vi "test_libssh2_userauth_publickey_fromfile.vi"() -> ()   [LabVIEW 2013, in "libssh2_integration_tests.lvlib"]
uses:
  libssh2_integration_tests.lvlib
  libssh2/libssh2_init_default.vi
  libssh2/libssh2_session_handshake_tcp.vi
  libssh2/libssh2.lvlib
  <vilib>/addons/_JKI Toolkits/Caraya/classes/Test/Test.lvclass
  <vilib>/addons/_JKI Toolkits/Caraya/classes/Assert/Assert.lvclass
panel:
  out "error out":errorcluster
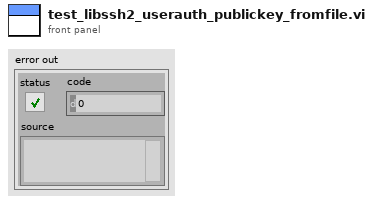
[diagram p1: front panel]
types:
  T1 = typedef "libssh2.lvlib/Session Refnum.ctl" = refnum<k1>
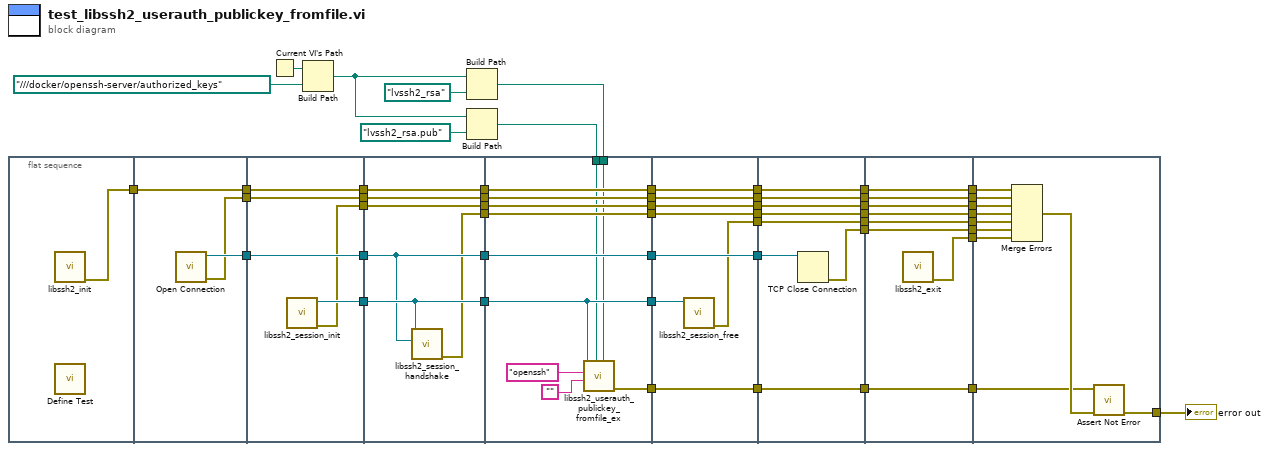
[diagram p0: block diagram]
diagram:
  n1 = flat-sequence {
    tunnel: [w53] -> w52
    tunnel: [w56] -> w51
    tunnel: w52 -> [w55]
    tunnel: [w55] -> w50
    tunnel: [w54] -> w49
    tunnel: w51 -> [w61]
    tunnel: [w61] -> w22
    tunnel: w50 -> [w60]
    tunnel: [w60] -> w21
    tunnel: w49 -> [w59]
    tunnel: [w59] -> w20
    tunnel: [w58] -> w19
    tunnel: [w57] -> w18
    tunnel: w22 -> [w63]
    tunnel: [w63] -> w37
    tunnel: w21 -> [w67]
    tunnel: [w67] -> w36
    tunnel: w20 -> [w66]
    tunnel: [w66] -> w35
    tunnel: [w65] -> w34
    tunnel: w19 -> [w65]
    tunnel: w18 -> [w64]
    tunnel: [w64] -> w33
    tunnel: [w62] -> w32
    tunnel: w37 -> [w78]
    tunnel: [w78] -> w14
    tunnel: w36 -> [w77]
    tunnel: [w77] -> w13
    tunnel: w35 -> [w76]
    tunnel: [w76] -> w12
    tunnel: w34 -> [w73]
    tunnel: w33 -> [w75]
    tunnel: [w75] -> w11
    tunnel: w32 -> [w74]
    tunnel: [w74] -> w10
    tunnel: [w73] -> w9
    tunnel: [w71] -> w8
    tunnel: w3 -> [w69]
    tunnel: w2 -> [w68]
    tunnel: w14 -> [w86]
    tunnel: [w86] -> w31
    tunnel: w13 -> [w85]
    tunnel: [w85] -> w30
    tunnel: w12 -> [w84]
    tunnel: [w84] -> w29
    tunnel: w11 -> [w83]
    tunnel: [w83] -> w28
    tunnel: w10 -> [w82]
    tunnel: [w82] -> w27
    tunnel: [w81] -> w24
    tunnel: [w80] -> w15
    tunnel: w8 -> [w80]
    tunnel: w9 -> [w79]
    tunnel: w31 -> [w94]
    tunnel: w30 -> [w93]
    tunnel: [w93] -> w48
    tunnel: w29 -> [w92]
    tunnel: [w92] -> w47
    tunnel: [w91] -> w46
    tunnel: w28 -> [w90]
    tunnel: [w90] -> w45
    tunnel: w27 -> [w89]
    tunnel: [w89] -> w44
    tunnel: [w88] -> w25
    tunnel: w24 -> [w88]
    tunnel: [w87] -> w16
    tunnel: w15 -> [w87]
    tunnel: w48 -> [w102]
    tunnel: [w102] -> w43
    tunnel: w47 -> [w101]
    tunnel: [w101] -> w42
    tunnel: w46 -> [w100]
    tunnel: [w100] -> w41
    tunnel: [w99] -> w40
    tunnel: w45 -> [w98]
    tunnel: [w98] -> w39
    tunnel: w44 -> [w97]
    tunnel: [w97] -> w38
    tunnel: [w96] -> w26
    tunnel: w25 -> [w96]
    tunnel: [w95] -> w17
    tunnel: w16 -> [w95]
    tunnel: w43 -> [w112]
    tunnel: w42 -> [w111]
    tunnel: w41 -> [w110]
    tunnel: w40 -> [w109]
    tunnel: w39 -> [w108]
    tunnel: [w106] -> w23
    tunnel: w38 -> [w105]
    tunnel: w26 -> [w104]
    tunnel: w17 -> [w103]
    frame #0 {
      n2 = call-poly "libssh2_init.vi"() -> ("error out"=w53:errorcluster)  [unwired: 11 in]
      n3 = call <vilib>:"Define Test.vi"() -> ()  [unwired: 10 in, 2 out]
    }
    frame #1 {
      n4 = call "Open Connection.vi"() -> ("error out"=w54:errorcluster, "connection ID"=w56:refnum<k5>)  [unwired: 10 in]
    }
    frame #2 {
      n5 = call "libssh2_session_init.vi"() -> ("error out"=w57:errorcluster, "session"=w58:T1)  [unwired: 10 in]
    }
    frame #3 {
      n6 = call-poly "libssh2_session_handshake.vi"("tcp connection"=w63, "session"=w65) -> ("error out"=w62:errorcluster)  [unwired: 9 in]
    }
    frame #4 {
      n7 = call "libssh2_userauth_publickey_fromfile_ex.vi"("private key"=w68, "public key"=w69, "passphrase"="", "username"="openssh", "session"=w73) -> ("error out"=w71:errorcluster)  [unwired: 6 in]
    }
    frame #5 {
      n8 = call "libssh2_session_free.vi"("session"=w79) -> ("error out"=w81:errorcluster)  [unwired: 10 in]
    }
    frame #6 {
      n9 = TCP Close Connection(connection ID=w94) -> (error out=w91:errorcluster)  [unwired: 2 in, 1 out]
    }
    frame #7 {
      n10 = call "libssh2_exit.vi"() -> ("error out"=w99:errorcluster)  [unwired: 11 in]
    }
    frame #8 {
      n11 = Merge Errors(w112, w111, w108, w105, w104, w110, w109) -> (w107:errorcluster)
      n12 = call <vilib>:"Assert Not Error.vi"("error in (no error)"=w107, "Not Error?"=w103) -> ("error out"=w106:errorcluster)  [unwired: 8 in, 1 out]
    }
  }
  n13 = Current VI's Path() -> (path=w1:path)
  n14 = Build Path(base path=w1, name or relative path=path "../../../docker/openssh-server/authorized_keys" ("stripped path")) -> (appended path=w4:path)
  n15 = Build Path(base path=w4, name or relative path=path "lvssh2_rsa" ("stripped path")) -> (appended path=w2:path)
  n16 = Build Path(base path=w4, name or relative path=path "lvssh2_rsa.pub" ("stripped path")) -> (appended path=w3:path)
  "error out" <- w23
